vi "01_强制类型转换DBL to I64.vi"() -> ()   [LabVIEW 2024]
doc: "本VI是为《我和LabVIEW》一书编写的示例。\n关于本书的介绍请参考网页：\nhttp://ruanqizhen.spaces.live.com/blog/cns!5852D4F797C53FB6!4310.entry"
panel:
  out "强制转换至类型":i64
  out "强制转类型转换函数":i64 format="%.0b"
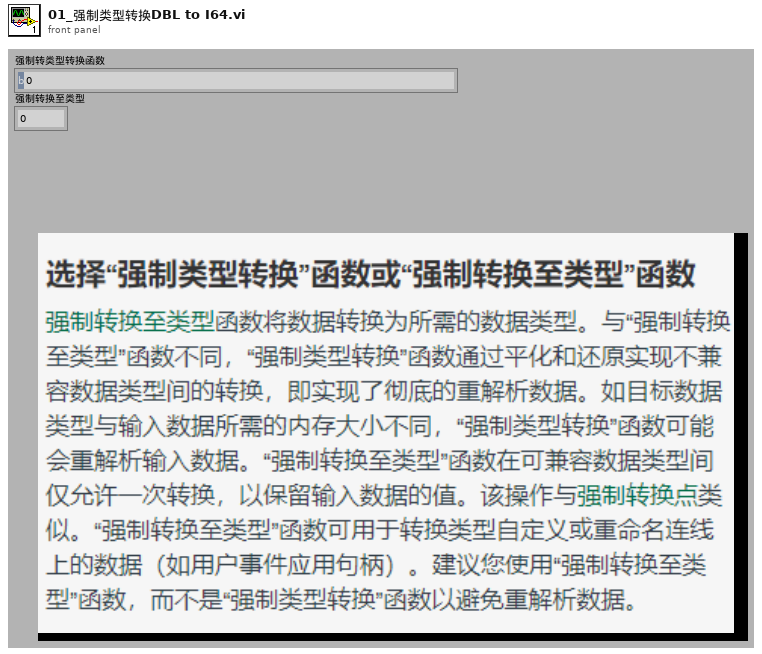
[diagram p1: front panel]
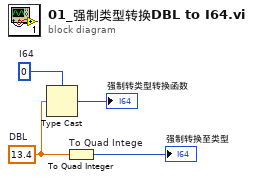
[diagram p0: block diagram]
diagram:
  w4 = i64 0  # I64
  w1 = 13.4  # DBL
  n1 = Type Cast(type=w4, x=w1) -> (*(type *) &x=→"强制转类型转换函数":i64)
  n2 = To Quad Integer "To Quad Intege"(1:w1) -> (0:→"强制转换至类型":i64)
